vi "Fpga main.vi"   [LabVIEW 2021]
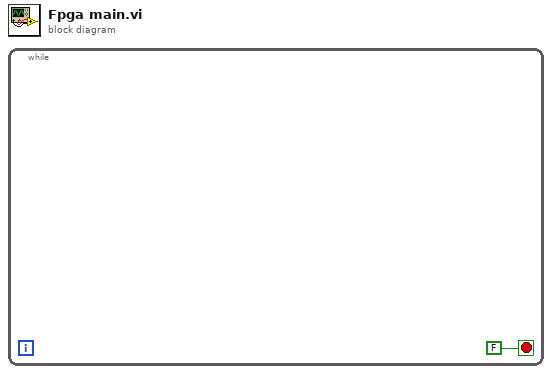
[diagram p0: block diagram]
diagram:
  n1 = while {
    stop <- FALSE stop-if-true
  }
